vi "test_rethinkdb_json_get.vi"() -> (0 "error out":errorcluster, 3 "all passed":bool)   [LabVIEW 2017]
uses:
  0448d06f-c907-48d3-8e95-609a58c9da34.vi
  6e78c047-ad8b-4c80-bf35-930779fc6639.vi
  adc0b81e-b473-424f-8777-4057b283b69f.vi
  fe157617-94d3-4ebf-b354-b7667e49f288.vi
  rethinkdb/json/json_resolve_key.vi
  rethinkdb/json/json_parse_value.vi
  rethinkdb/json/json_cache.vi
panel:
  out "passed":bool[](array[boolean])
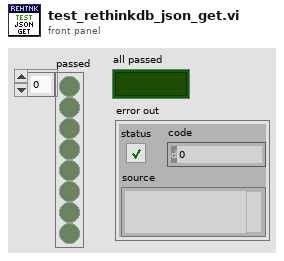
[diagram p1: front panel]
types:
  T1 = typedef "json_element.ctl" = cluster{"path":string, "type":T2, "value":variant}
  T2 = typedef "json_element_type.ctl" = enum8{"null", "bool", "int", "uint", "float", "string", "array", "object"}
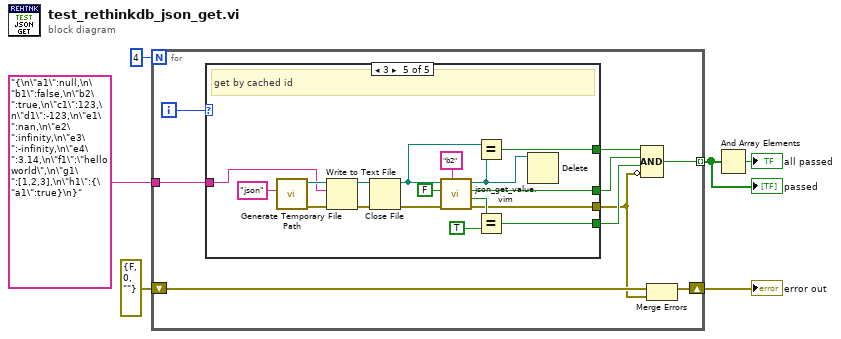
[diagram p0: block diagram]
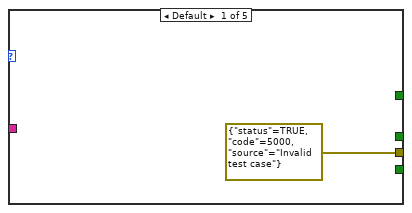
[diagram p2: hidden frame]
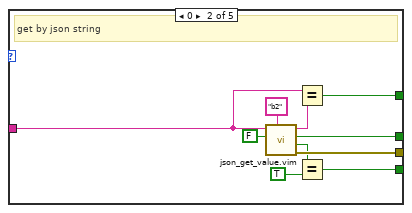
[diagram p3: hidden frame]
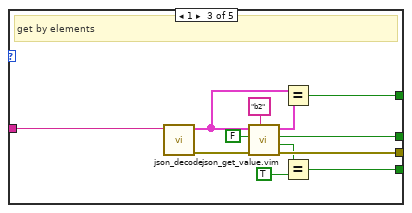
[diagram p4: hidden frame]
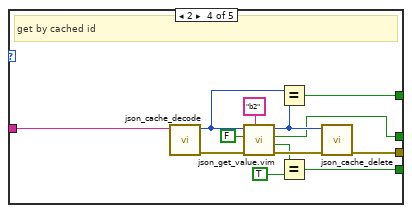
[diagram p5: hidden frame]
diagram:
  n1 = for {
    N: 4 -> [_]
    tunnel: [w10] -> w6 mode=indexing
    tunnel: "{\n\"a1\":null,\n\"b1\":false,\n\"b2\":true,\n\"c1\":123,\n\"d1\":-123,\n\"e1\":nan,\n\"e2\":infinity,\n\"e3\":-infinity,\n\"e4\":3.14,\n\"f1\":\"hello world\",\n\"g1\":[1,2,3],\n\"h1\":{\"a1\":true}\n}" ("json") -> [w15]
    shift-right: [w7] -> w1
    shift-left: errorcluster {"status"=FALSE, "code"=0, "source"=""} ("error in (no error)") -> [w9]
    i -> [w14]
    n2 = case shown="3" w14 {
      tunnel: [_ w23 w33 w40 w63] -> w12
      tunnel: [errorcluster {"status"=TRUE, "code"=5000, "source"="Invalid test case"} ("error out") w24 w34 w47 w57] -> w8
      tunnel: w15 -> [_ w22 w36 w46 w54]
      tunnel: [_ w18 w28 w41 w64] -> w13
      tunnel: [_ w17 w27 w39 w62] -> w11
      frame Default {
      }
      frame 0 {
        # "get by json string"
        n3 = call "json_get_value.vim"("key"="b2", "default"=FALSE, "elements in"=w22) -> ("error out"=w24:errorcluster, "exists?"=w20:bool, "value"=w23:bool, "elements out"=w21:string)  [unwired: 5 in]
        n4 = Equal?(x=w22, y=w21) -> (x = y?=w18:bool)
        n5 = Equal?(x=w20, y=TRUE) -> (x = y?=w17:bool)
      }
      frame 1 {
        # "get by elements"
        n6 = call "json_decode.vi"("json"=w36) -> ("error out"=w35:errorcluster, "elements"=w31:T1[])  [unwired: 9 in]
        n7 = call "json_get_value.vim"("key"="b2", "error in (no error)"=w35, "default"=FALSE, "elements in"=w31) -> ("error out"=w34:errorcluster, "exists?"=w30:bool, "value"=w33:bool, "elements out"=w32:T1[])  [unwired: 4 in]
        n8 = Equal?(x=w31, y=w32) -> (x = y?=w28:bool)
        n9 = Equal?(x=w30, y=TRUE) -> (x = y?=w27:bool)
      }
      frame 2 {
        # "get by cached id"
        n10 = call "json_cache_decode.vi"("json"=w46) -> ("error out"=w51:errorcluster, "cache id"=w44:u64)  [unwired: 9 in]
        n11 = call "json_get_value.vim"("key"="b2", "error in (no error)"=w51, "default"=FALSE, "elements in"=w44) -> ("error out"=w48:errorcluster, "exists?"=w43:bool, "value"=w40:bool, "elements out"=w45:u64)  [unwired: 4 in]
        n12 = Equal?(x=w44, y=w45) -> (x = y?=w41:bool)
        n13 = Equal?(x=w43, y=TRUE) -> (x = y?=w39:bool)
        n14 = call "json_cache_delete.vi"("error in (no error)"=w48, "cache id"=w45) -> ("error out"=w47:errorcluster)  [unwired: 7 in, 2 out]
      }
      frame 3 {
        # "get by cached id"
        n15 = call <vilib>:"Generate Temporary File Path.vi"("Temporary File Extension (tmp)"="json") -> ("error out"=w56:errorcluster, "Unique Temporary File Path"=w55:path)  [unwired: 9 in]
        n16 = Write to Text File(file (use dialog)=w55, text=w54, error in=w56) -> (refnum out=w60:refnum<file>, error out=w61:errorcluster)  [unwired: 1 in, 1 out]
        n17 = Close File(refnum=w60, error in=w61) -> (path=w58:path, error out=w59:errorcluster)
        n18 = call "json_get_value.vim"("key"="b2", "error in (no error)"=w59, "default"=FALSE, "elements in"=w58) -> ("error out"=w57:errorcluster, "exists?"=w66:bool, "value"=w63:bool, "elements out"=w53:path)  [unwired: 4 in]
        n19 = Equal?(x=w58, y=w53) -> (x = y?=w64:bool)
        n20 = Equal?(x=w66, y=TRUE) -> (x = y?=w62:bool)
        n21 = Delete(path (use dialog)=w53) -> ()  [unwired: 4 in, 3 out]
      }
    }
    n22 = Compound Arithmetic op=AND(w13, w12, w11, invert w8) -> (w10:bool)
    n23 = Merge Errors(w9, w8) -> (w7:errorcluster)
  }
  "error out" <- w1
  "passed" <- w6
  n24 = And Array Elements(Boolean array=w6) -> (logical AND=→"all passed":bool)
